vi "sub_encode_credentials.vi"(7 "Command":T1, 8 "error in":errorcluster, 9 "line separator (\\n)":string="\n", 10 "Password":string, 11 "User Name":string) -> (0 "error out":errorcluster, 2 "Stored Credentials":string, 3 "Credentials":string)   [LabVIEW 2013, in "daqio minimal.lvlib"]
doc: "This VI encodes user credentials and keeps them available in an FGV."
uses:
  daqio minimal.lvlib
  _typedefs/daqio-Credentials-FGV.ctl
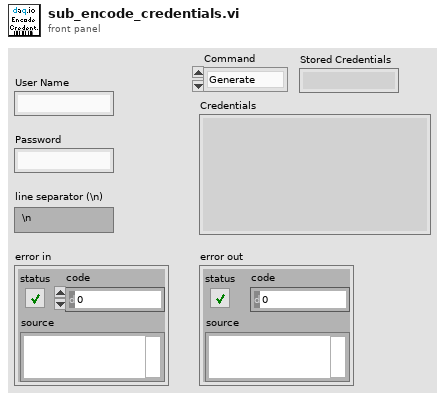
[diagram p1: front panel]
types:
  T1 = typedef "daqio minimal.lvlib/daqio-Credentials-FGV.ctl" = enum16{"Generate", "Read"}
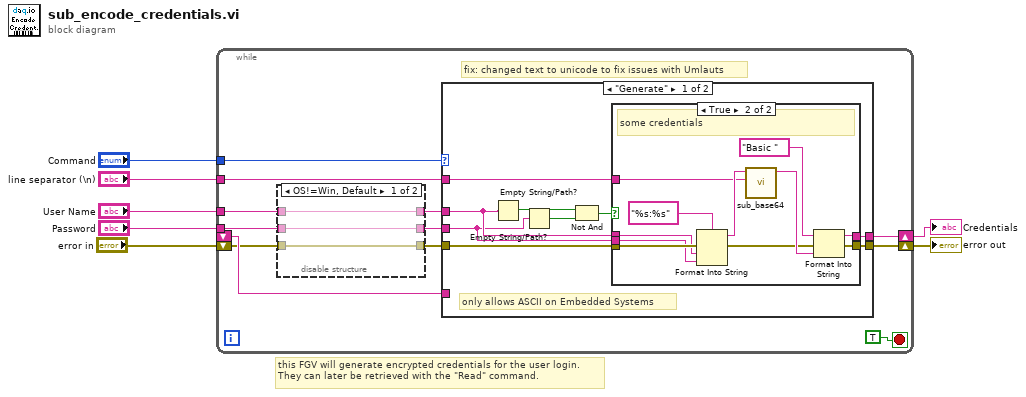
[diagram p0: block diagram]
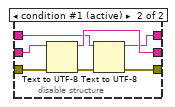
[diagram p2: hidden frame]
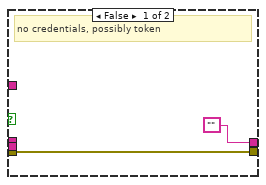
[diagram p3: hidden frame]
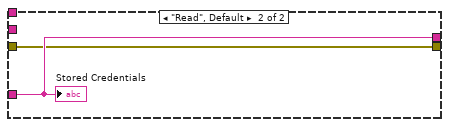
[diagram p4: hidden frame]
diagram:
  # "this FGV will generate encrypted credentials for the user login.\nThey can later be retrieved with the \"Read\" command."
  n1 = while {
    tunnel: "line separator (\\n)" -> [w19]
    tunnel: "Password" -> [w11]
    tunnel: "User Name" -> [w13]
    shift-right: [w18] -> w5
    shift-left: "error in" -> [w9]
    shift-right: [w17] -> w4
    shift-left: _ -> [w14]
    tunnel: "Command" -> [w15]
    stop <- TRUE stop-if-true
    # "fix: changed text to unicode to fix issues with Umlauts"
    n2 = disable-structure shown="OS!=Win, Default" {
      disable-tunnel: w13 -> [w21 w24]
      disable-tunnel: [w21 w23] -> w12
      disable-tunnel: w11 -> [w20 w26]
      disable-tunnel: [w20 w25] -> w10
      disable-tunnel: w9 -> [w22 w28]
      disable-tunnel: [w22 w27] -> w8
      frame condition #0 {
      }
      frame condition #1 (active) {
        n3 = Text to UTF-8(8:w28, 11:w26) -> (0:w29:errorcluster, 3:w25:string)
        n4 = Text to UTF-8(8:w29, 11:w24) -> (0:w27:errorcluster, 3:w23:string)
      }
    }
    n5 = case shown="\"Generate\"" w15 {
      tunnel: w19 -> [w38 _]
      tunnel: w8 -> [w37 w52]
      tunnel: [w36 w52] -> w18
      tunnel: [w35 w53] -> w17
      tunnel: w10 -> [w33 _]
      tunnel: w12 -> [w34 _]
      tunnel: w14 -> [_ w53]
      frame "Generate" {
        # "only allows ASCII on Embedded Systems"
        n6 = Empty String/Path?(string/path=w34) -> (empty?=w32:bool)
        n7 = Empty String/Path?(string/path=w33) -> (empty?=w31:bool)
        n8 = Not And(1:w31, 2:w32) -> (0:w30:bool)
        n9 = case shown="True" w30 {
          tunnel: w38 -> [_ w49]
          tunnel: w37 -> [w39 w48]
          tunnel: [w39 w47] -> w36
          tunnel: ["" w46] -> w35
          tunnel: w34 -> [_ w42]
          tunnel: w33 -> [_ w41]
          frame False {
            # "no credentials, possibly token"
          }
          frame True {
            # "some credentials"
            n10 = Format Into String(format string="%s:%s" ("Command"), error in=w48, w42, w41) -> (resulting string=w50:string, error out=w43:errorcluster)  [unwired: 1 in]
            n11 = call "sub_base64.vi"("line separator (\\n)"=w49, "String in"=w50) -> ("String out"=w51:string)  [unwired: 9 in]
            n12 = Format Into String(initial string="Basic " ("Command"), error in=w43, w51) -> (resulting string=w46:string, error out=w47:errorcluster)  [unwired: 1 in]
          }
        }
      }
      frame "Read", Default {
        "Stored Credentials" <- w53
      }
    }
  }
  "error out" <- w5
  "Credentials" <- w4
